vi "Rumble.vi"(8 "/limelight/tx":dbl, 9 "auto align (t/f)":bool, 10 "JoystickDevRef 1":T1, 11 "JoystickDevRef 0":T1) -> ()   [LabVIEW 2020]
uses:
  <vilib>/Rock Robotics/WPI/Joystick/WPI_JoystickDevRef.ctl
  <vilib>/Rock Robotics/WPI/Joystick/WPI_JoystickDeviceEnum.ctl
panel:
  out "Numeric":dbl
  in  "epoxy left":dbl=0.050000000000000044 format="%#_13g"
  in  "epoxy right":dbl=0.3 format="%#_13g"
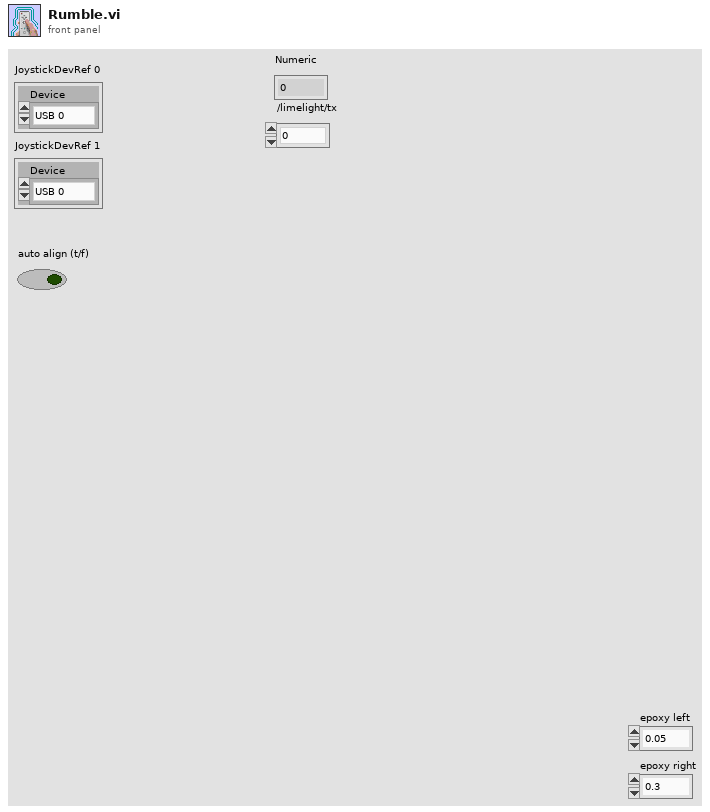
[diagram p1: front panel]
types:
  T1 = typedef "WPI_JoystickDevRef.ctl" = cluster{"Device":T2}
  T2 = typedef "WPI_JoystickDeviceEnum.ctl" = enum16{"USB 0", "USB 1", "USB 2", "USB 3", "USB 4", "USB 5"}
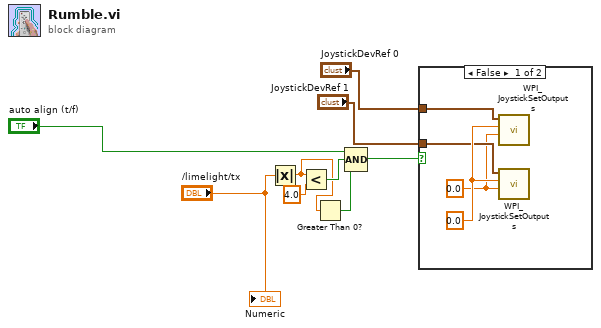
[diagram p0: block diagram]
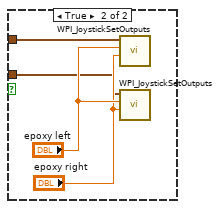
[diagram p2: hidden frame]
diagram:
  n1 = Absolute Value(x="/limelight/tx") -> (abs(x)=w6:dbl)
  n2 = Less?(x=w6, y=4.0) -> (x < y?=w7:bool)
  n3 = Greater Than 0?(x=w6) -> (x > 0?=w5:bool)
  n4 = Compound Arithmetic op=AND("auto align (t/f)", w7, w5) -> (w8:bool)
  n5 = case shown="False" w8 {
    tunnel: "JoystickDevRef 0" -> [w12 w15]
    tunnel: "JoystickDevRef 1" -> [w11 w14]
    frame False {
      w10 = sgl 0.0 ("Right Rumble")
      w13 = sgl 0.0 ("Left Rumble")
      n6 = call <vilib>:"WPI_JoystickSetOutputs.vi"("Right Rumble"=w10, "Left Rumble"=w13, "JoystickDevRef"=w12) -> ()  [unwired: 7 in, 2 out]
      n7 = call <vilib>:"WPI_JoystickSetOutputs.vi"("Right Rumble"=w10, "Left Rumble"=w13, "JoystickDevRef"=w11) -> ()  [unwired: 7 in, 2 out]
    }
    frame True {
      n8 = call <vilib>:"WPI_JoystickSetOutputs.vi"("Right Rumble"="epoxy right", "Left Rumble"="epoxy left", "JoystickDevRef"=w15) -> ()  [unwired: 7 in, 2 out]
      n9 = call <vilib>:"WPI_JoystickSetOutputs.vi"("Right Rumble"="epoxy right", "Left Rumble"="epoxy left", "JoystickDevRef"=w14) -> ()  [unwired: 7 in, 2 out]
    }
  }
  "Numeric" <- "/limelight/tx"
